vi "Build Package Cmd.vi"(0 "Source Path":path, 5 "Destination Dir":path, 11 "error in (no error)":errorcluster) -> (4 "Error Message":string, 15 "error out":errorcluster)   [LabVIEW 2021, in "Packager Helpers.lvlib"]
uses:
  Packager Helpers.lvlib
  Path Functions/Path Functions.lvlib
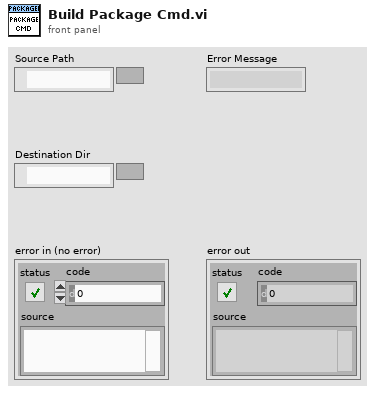
[diagram p1: front panel]
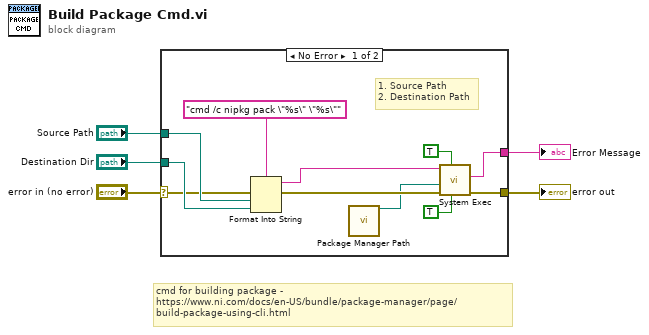
[diagram p0: block diagram]
diagram:
  # "cmd for building package -\nhttps://www.ni.com/docs/en-US/bundle/package-manager/page/build-package-using-cli.html"
  n1 = case shown="No Error" "error in (no error)" {
    selector: "error in (no error)" -> [w9 w17]
    tunnel: [w6 w17] -> w5
    tunnel: "Destination Dir" -> [w16 _]
    tunnel: "Source Path" -> [w15 _]
    tunnel: [w8 _] -> w2
    frame No Error {
      # "1. Source Path\n2. Destination Path"
      n2 = Format Into String(format string="cmd /c nipkg pack \"%s\" \"%s\"", error in=w9, w15, w16) -> (resulting string=w14:string, error out=w10:errorcluster)  [unwired: 1 in]
      n3 = call "Package Manager Path.vi"() -> ("Package Manager Path"=w7:path)  [unwired: 15 in]
      n4 = call <vilib>:"System Exec.vi"("run minimized? (F)"=TRUE, "wait until completion? (T)"=TRUE, "error in (no error)"=w10, "working directory"=w7, "command line"=w14) -> ("error out"=w6:errorcluster, "standard error"=w8:string)  [unwired: 3 in, 2 out]
    }
    frame Error {
    }
  }
  "error out" <- w5
  "Error Message" <- w2
